vi "SetBuiltOnError.vi"(8 "error in (no error)":errorcluster, 11 "ProjectItem in":refnum<class "ProjectItem.lvclass">) -> (0 "error out":errorcluster, 3 "ProjectItem out":refnum<class "ProjectItem.lvclass">)   [LabVIEW 2019, in "SolutionBuilder.lvlib" / "ProjectItem.lvclass"]
uses:
  ProjectItem.lvclass
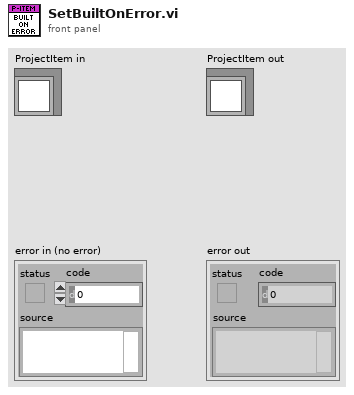
[diagram p1: front panel]
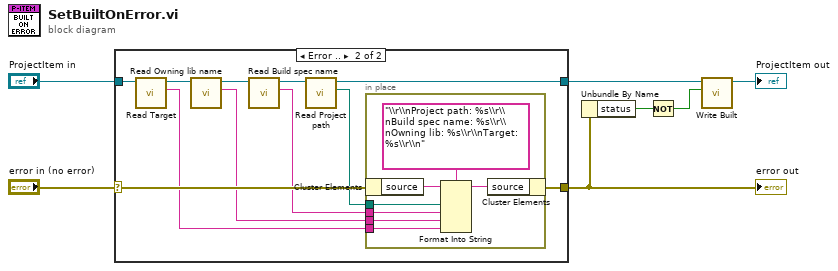
[diagram p0: block diagram]
diagram:
  n1 = case shown="Error .." "error in (no error)" {
    selector: "error in (no error)" -> [w8 w20]
    tunnel: "ProjectItem in" -> [w9 w12]
    tunnel: [w9 w16] -> w2
    tunnel: [w8 w19] -> w1
    frame No Error {
    }
    frame Error {
      n2 = call "Read Target.vi"("ProjectItem in"=w12) -> ("Target"=w10:string, "ProjectItem out"=w11:refnum<class "ProjectItem.lvclass">)  [unwired: 9 in]
      n3 = call "Read Owning lib name.vi"("ProjectItem in"=w11) -> ("Owning lib name"=w15:string, "ProjectItem out"=w18:refnum<class "ProjectItem.lvclass">)  [unwired: 9 in]
      n4 = call "Read Build spec name.vi"("ProjectItem in"=w18) -> ("Build spec name"=w14:string, "ProjectItem out"=w17:refnum<class "ProjectItem.lvclass">)  [unwired: 9 in]
      n5 = call "Read Project path.vi"("ProjectItem in"=w17) -> ("Project path"=w13:path, "ProjectItem out"=w16:refnum<class "ProjectItem.lvclass">)  [unwired: 9 in]
      n6 = in-place {
        in-place-border: w15 -> [w24]
        in-place-border: w14 -> [w23]
        in-place-border: w13 -> [w22]
        in-place-border: w10 -> [w21]
        n7 = in-place-cluster #1(w20) -> ("source"=w27:string)
        n8 = Format Into String(format string="\\r\\nProject path: %s\\r\\nBuild spec name: %s\\r\\nOwning lib: %s\\r\\nTarget: %s\\r\\n", initial string=w27, w22, w23, w24, w21) -> (resulting string=w25:string)  [unwired: 1 in, 1 out]
        n9 = in-place-cluster #1("source"=w25) -> (w19:errorcluster)
      }
    }
  }
  "error out" <- w1
  n10 = Unbundle By Name(w1) -> ("status"=w6:bool)
  n11 = Not(x=w6) -> (.not. x?=w5:bool)
  n12 = call "Write Built.vi"("Built"=w5, "ProjectItem in"=w2) -> ("ProjectItem out"=→"ProjectItem out":refnum<class "ProjectItem.lvclass">)  [unwired: 9 in]
